vi "get crate map lecroy.vi"(0 "VISA In":refnum<visa-resource-name>, 3 "Crate":i32, 5 "error in":errorcluster) -> (14 "VISA out":refnum<visa-resource-name>, 16 "Crate Details":T1, 19 "error out":errorcluster)   [LabVIEW 2018]
uses:
  crate.ctl
  card.ctl
  Tom Shaw/Lecroy Control/HV Documentation and Software for Testing/SubVIs/General_lecroy_command.ctl
  CAEN globals.vi
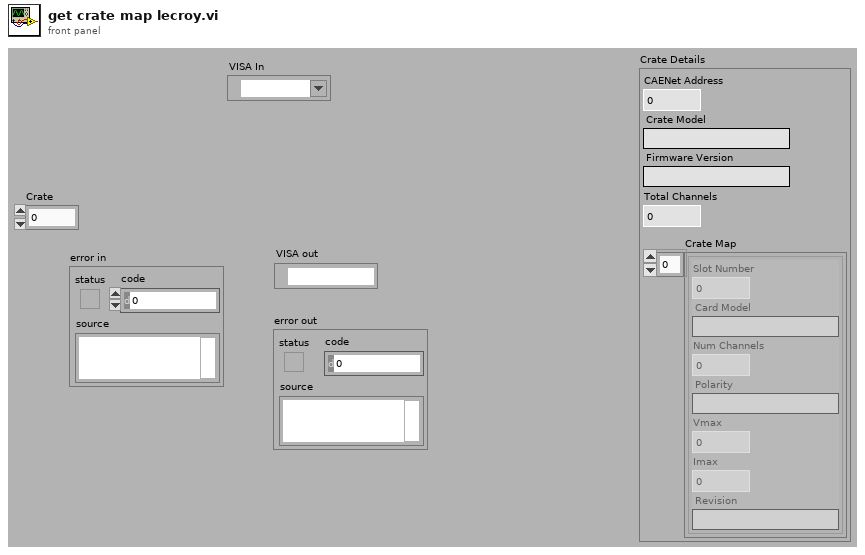
[diagram p1: front panel]
types:
  T1 = typedef "crate.ctl" = cluster{"CAENet Address":i32, "Crate Model":string, "Firmware Version":string, "Crate Map":T2[], "Total Channels":i32}
  T2 = typedef "card.ctl" = cluster{"Slot Number":i32, "Card Model":string, "Num Channels":i32, "Polarity":string, "Vmax":dbl, "Imax":dbl, "Revision":string}
  T3 = enum16{"Monitor", "Demand", "Backup", "All", "None"}
  T4 = typedef "General_lecroy_command.ctl" = string
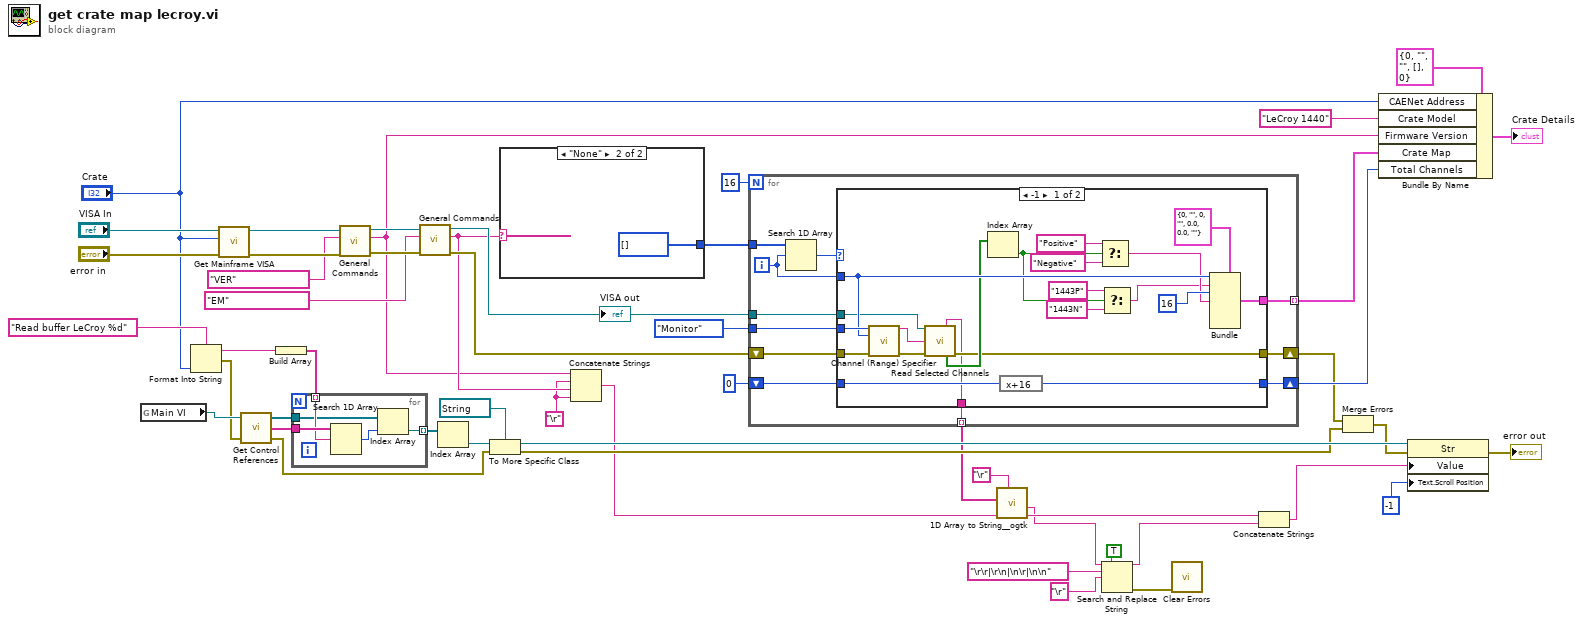
[diagram p0: block diagram]
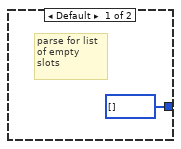
[diagram p2: hidden frame]
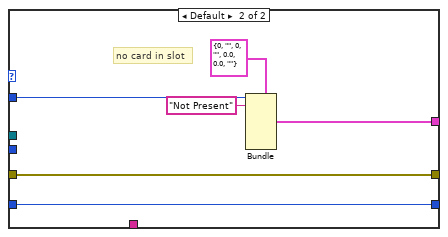
[diagram p3: hidden frame]
diagram:
  w11 = "\r"
  n1 = global read "CAEN globals.vi" "Main VI"() -> (w28:refnum<vi>)
  n2 = Format Into String(format string="Read buffer LeCroy %d" ("Label.Text"), "Crate") -> (resulting string=w22:string, error out=w23:errorcluster)  [unwired: 2 in]
  n3 = call "Get Mainframe VISA.vi"("Error In"="error in", "Crate"="Crate", "VISA In"="VISA In") -> ("Error Out"=w46:errorcluster, "VISA out"=w47:refnum<visa-resource-name>)  [unwired: 6 in, 1 out]
  n4 = call "Get Control References.vi"("error in"=w23, "This vi"=w28) -> ("error out"=w25:errorcluster, "Control Names"=w29:string[], "Controls[]"=w30:refnum<vi>[])  [unwired: 1 in]
  n5 = Build Array(w22) -> (w24:string[])
  n6 = for {
    tunnel: w29 -> [w55]
    tunnel: w24 -> [w54] mode=indexing
    tunnel: w30 -> [w53]
    tunnel: [w52] -> w31 mode=indexing
    n7 = Search 1D Array(1D array=w55, element=w54) -> (index of element=w51:i32)  [unwired: 1 in]
    n8 = Index Array(array=w53, index=w51) -> (element=w52:refnum<vi>)
  }
  n9 = call "General Commands.vi"("error in"=w46, "Action"=T4 "VER", "VISA in"=w47) -> ("error out"=w43:errorcluster, "result string"=w12:string, "VISA out"=w44:refnum<visa-resource-name>)  [unwired: 6 in]
  n10 = call "General Commands.vi"("error in"=w43, "Action"=T4 "EM", "VISA in"=w44) -> ("error out"=w36:errorcluster, "result string"=w13:string, "VISA out"=w34:refnum<visa-resource-name>)  [unwired: 6 in]
  "VISA out" <- w34
  n11 = Index Array(array=w31) -> (element=w26:refnum<vi>)  [unwired: 1 in]
  n12 = To More Specific Class(target class=refnum<vi> refnum ("s? t:f"), reference=w26, error in=w25) -> (specific class reference=w17:refnum<vi>, error out=w15:errorcluster)
  n13 = case shown="\"None\"" w13 {
    tunnel: [i32[] [] i32[] []] -> w39
    frame Default {
      # "parse for list\nof empty \nslots"
    }
    frame "None" {
    }
  }
  n14 = Concatenate Strings(w12, w11, w13, w11) -> (w7:string)
  n15 = for {
    N: 16 -> [_]
    tunnel: [w68] -> w41 mode=indexing
    shift-right: [w63] -> w38
    shift-left: 0 ("Slot Number") -> [w64]
    tunnel: w39 -> [w67]
    shift-right: [w59] -> w16
    shift-left: w36 -> [w62]
    tunnel: T3."Monitor" ("Buffer") -> [w61]
    tunnel: w34 -> [w60]
    tunnel: [w58] -> w10 mode=indexing
    i -> [w65]
    n16 = Search 1D Array(1D array=w67, element=w65) -> (index of element=w66:i32)  [unwired: 1 in]
    n17 = case shown="-1" w66 {
      tunnel: [w88 w94] -> w68
      tunnel: w65 -> [w82 w93]
      tunnel: w64 -> [w86 w92]
      tunnel: [w87 w92] -> w63
      tunnel: w62 -> [w84 w90]
      tunnel: w61 -> [w83 _]
      tunnel: w60 -> [w81 _]
      tunnel: [w74 w90] -> w59
      tunnel: [w73 _] -> w58
      frame -1 {
        n18 = call "Channel (Range) Specifier.vi"("Buffer"=w83, "Card"=w82, "error in"=w84) -> ("Channel (Range)"=w79:string, "error out"=w80:errorcluster)  [unwired: 11 in]
        n19 = call "Read Selected Channels.vi"("VISA in"=w81, "C##,##DO###"=w79, "error in"=w80) -> ("Final Output"=w73:string, "Channel Polarity (T: Negative, F: Positive)"=w75:bool[], "error out"=w74:errorcluster)  [unwired: 6 in, 4 out]
        n20 = Index Array(array=w75) -> (element=w69:bool)  [unwired: 1 in]
        n21 = expression code="x+16"(w86) -> (w87:i32)
        n22 = Select(t="Positive" ("x"), s=w69, f="Negative" ("x")) -> (s? t:f=w78:string)
        n23 = Select(t="1443P" ("x"), s=w69, f="1443N" ("x")) -> (s? t:f=w70:string)
        n24 = Bundle(cluster=T2 {"Slot Number"=0, "Card Model"="", "Num Channels"=0, "Polarity"="", "Vmax"=0.0, "Imax"=0.0, "Revision"=""} ("output cluster"), "Slot Number"=w82, "Card Model"=w70, "Num Channels"=16, "Polarity"=w78) -> (w88:T2)  [unwired: 3 in]
      }
      frame Default {
        # "no card in slot"
        n25 = Bundle(cluster=T2 {"Slot Number"=0, "Card Model"="", "Num Channels"=0, "Polarity"="", "Vmax"=0.0, "Imax"=0.0, "Revision"=""} ("output cluster"), "Slot Number"=w93, "Card Model"="Not Present") -> (w94:T2)  [unwired: 5 in]
      }
    }
  }
  n26 = call <userlib>:"1D Array to String__ogtk.vi"("delimiter (Tab)"="\r", "Array of Strings"=w10) -> ("delimited string"=w2:string)  [unwired: 9 in]
  n27 = Search and Replace String(replace all?=TRUE ("replace all? (F)"), input string=w2, search string="\r\r|\r\n|\n\r|\n\n", replace string="\r" ("search string")) -> (result string=w1:string, error out=w3:errorcluster)  [unwired: 4 in, 2 out]
  n28 = call <vilib>:"Clear Errors.vi"("error in (no error)"=w3) -> ()  [unwired: 5 in, 2 out]
  n29 = Concatenate Strings(w7, w1) -> (w8:string)
  n30 = Merge Errors(w16, w15) -> (w14:errorcluster)
  n31 = Bundle By Name(cluster=T1 {"CAENet Address"=0, "Crate Model"="", "Firmware Version"="", "Crate Map"=[], "Total Channels"=0} ("output cluster"), "CAENet Address"="Crate", "Crate Model"="LeCroy 1440" ("result string"), "Firmware Version"=w12, "Crate Map"=w41, "Total Channels"=w38) -> (→"Crate Details":T1)
  n32 = property class="Str"(reference=w17, error in=w14, "Value"=w8, "Text.Scroll Position"=-1) -> (error out=→"error out":errorcluster)  [unwired: 1 out]
